vi "Get Buffer Length.vi"(8 "error in (no error)":errorcluster, 9 "Buffer Name ()":string, 11 "VISA resource name":refnum<visa-resource-name>) -> (0 "error out":errorcluster, 2 "Buffer Count":i32, 3 "VISA resource name out":refnum<visa-resource-name>)   [LabVIEW 2023, in "Keithley DMM6500 DAQ6500 Series.lvlib"]
doc: "Reads and returns the buffer size specified by the Buffer Name."
uses:
  <instrlib>/Keithley DMM6500 DAQ6500 Series/Keithley DMM6500 DAQ6500 Series.lvlib
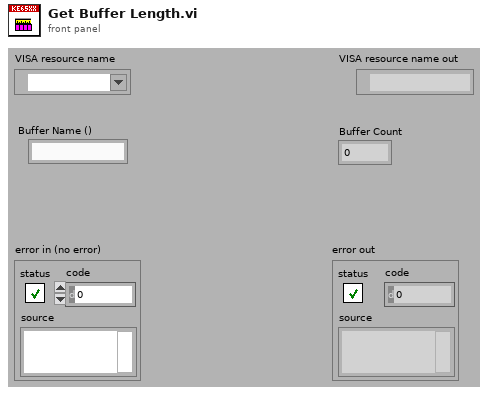
[diagram p1: front panel]
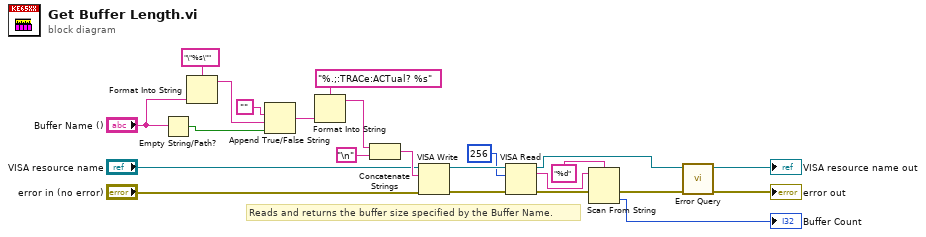
[diagram p0: block diagram]
diagram:
  # "Reads and returns the buffer size specified by the Buffer Name."
  n1 = Empty String/Path?(string/path="Buffer Name ()") -> (empty?=w1:bool)
  n2 = Format Into String(format string="\"%s\"", "Buffer Name ()") -> (resulting string=w10:string)  [unwired: 2 in, 1 out]
  n3 = Append True/False String(1:w1, 2:w10, 3:"") -> (0:w20:string)  [unwired: 1 in]
  n4 = Format Into String(format string="%.;:TRACe:ACTual? %s", w20) -> (resulting string=w17:string)  [unwired: 2 in, 1 out]
  n5 = Concatenate Strings(w17, "\n") -> (w19:string)
  n6 = VISA Write(VISA resource name="VISA resource name", write buffer=w19, error in (no error)="error in (no error)") -> (VISA resource name out=w14:refnum<visa-resource-name>, error out=w13:errorcluster)  [unwired: 1 out]
  n7 = VISA Read(VISA resource name=w14, byte count=u32 256, error in (no error)=w13) -> (VISA resource name out=w4:refnum<visa-resource-name>, read buffer=w8:string, error out=w11:errorcluster)  [unwired: 1 out]
  n8 = Scan From String(format string="%d", input string=w8, error in=w11) -> (error out=w5:errorcluster, output 1=→"Buffer Count":i32)  [unwired: 2 in, 2 out]
  n9 = call <instrlib>:"Error Query.vi"("error in (no error)"=w5, "VISA resource name"=w4) -> ("error out"=→"error out":errorcluster, "VISA resource name out"=→"VISA resource name out":refnum<visa-resource-name>)  [unwired: 6 in, 2 out]
